vi "Water Level Detector.vi"() -> ()   [LabVIEW 2020]
panel:
  out "Report":string
  out "Water Level is lower":bool
  out "Water Level is higher":bool
  out "Water Lever":u8(slide) scale=0.0..100.0
  in  "Water Tanker":dbl(slide) scale=0.0..100.0
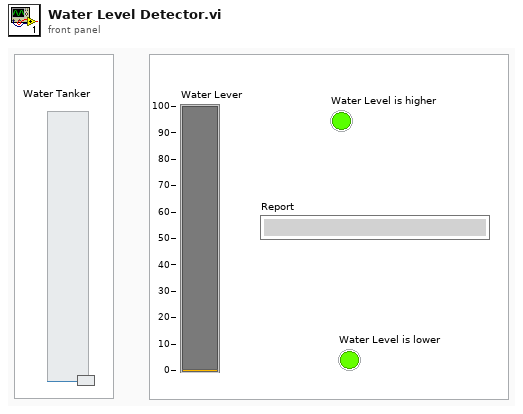
[diagram p1: front panel]
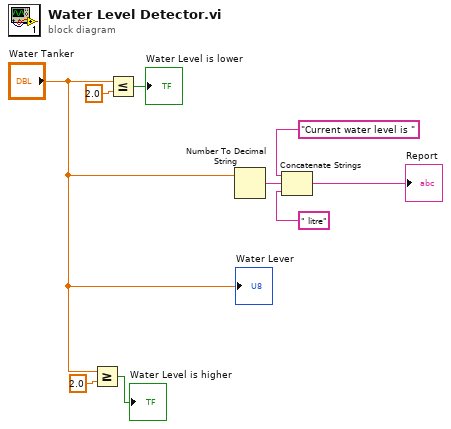
[diagram p0: block diagram]
diagram:
  n1 = Greater Or Equal?(x="Water Tanker", y=2.0) -> (x >= y?=→"Water Level is higher":bool)
  n2 = Less Or Equal?(x="Water Tanker", y=2.0) -> (x <= y?=→"Water Level is lower":bool)
  n3 = Number To Decimal String(number="Water Tanker") -> (decimal integer string=w4:string)  [unwired: 1 in]
  n4 = Concatenate Strings "Concatenate Strings"("Current water level is ", w4, " litre") -> (→"Report":string)
  "Water Lever" <- "Water Tanker"
